vi "Smart Open.vi"(7 "Allow multiple opens?":bool=TRUE, 8 "error in (no error)":errorcluster, 10 "Channel Names":tag[](array[tag])) -> (0 "error out":errorcluster, 3 "DIO Ref Out":T1)   [LabVIEW 2021, in "DIO.lvlib"]
uses:
  <vilib>/myRIO/Instrument Drivers/Onboard IO/DIO/DIO.lvlib
  <vilib>/myRIO/Common/Instrument Driver Framework/Utilities/typedefs/Hardware Version Enum.ctl
  <vilib>/myRIO/Common/Instrument Driver Framework/Utilities/typedefs/Generic FPGA Reference.ctl
  <vilib>/myRIO/Common/Instrument Driver Framework/myRIO v1.0/DIO/typedefs/DIO Channels Enum.ctl
  <vilib>/myRIO/Common/Instrument Driver Framework/myRIO v1.0/DIO/typedefs/DIO Channels List.ctl
  <vilib>/myRIO/Instrument Drivers/Onboard IO/DIO/typedefs/DIO Reference.ctl
  <vilib>/myRIO/Common/Instrument Driver Framework/Utilities/typedefs/myRIO v1.0 Reference.ctl
  <vilib>/myRIO/Common/Instrument Driver Framework/Utilities/typedefs/myRIO Generic Hardware Reference.ctl
  <vilib>/myRIO/Instrument Drivers/Onboard IO/DIO/vis/myRIO DIO Open.xnode
  <vilib>/myRIO/Common/Instrument Driver Framework/myRIO v1.0/DIO/vis/myRIO v1.1 Open DIO.vi
  <vilib>/userdefined/High Color/nirio_resource_hc.ctl
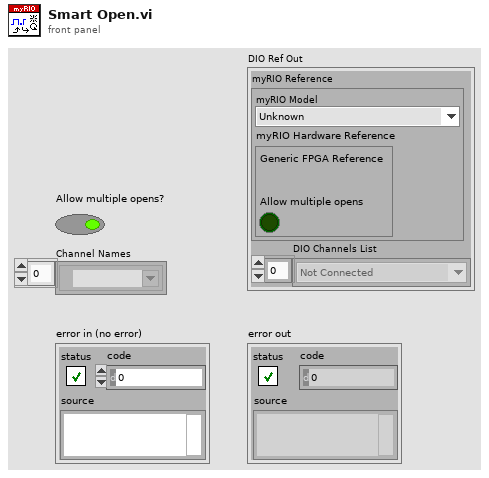
[diagram p1: front panel]
types:
  T1 = typedef "DIO.lvlib/DIO Reference.ctl" = cluster{"myRIO Reference":T2, "DIO Channels List":T6}
  T2 = typedef "myRIO Generic Hardware Reference.ctl" = cluster{"myRIO Model":T3, "myRIO Hardware Reference":T4}
  T3 = typedef "Hardware Version Enum.ctl" = enum16{"Unknown", "myRIO-1900", "myRIO-1950", "roboRIO", "NI ELVIS RIO CM", "ELVIS III"}
  T4 = typedef "myRIO v1.0 Reference.ctl" = cluster{"Generic FPGA Reference":T5, "Allow multiple opens":bool}
  T5 = typedef "Generic FPGA Reference.ctl" = refnum<k20>
  T6 = typedef "DIO Channels List.ctl" = T7[]
  T7 = typedef "DIO Channels Enum.ctl" = enum16{"Not Connected", "C/DIO0", "C/DIO1", "C/DIO2", "C/DIO3", "C/DIO4", "C/DIO5", "C/DIO6", "C/DIO7", "A/DIO0", "A/DIO1", "A/DIO2", "A/DIO3", "A/DIO4", "A/DIO5", "A/DIO6", "A/DIO7", "A/DIO8", "A/DIO9", "A/DIO10", "A/DIO11", "A/DIO12", "A/DIO13", "A/DIO14", "A/DIO15", "A/DIO16", "A/DIO17", "A/DIO18", "A/DIO19", "B/DIO0", "B/DIO1", "B/DIO2", "B/DIO3", "B/DIO4", "B/DIO5", "B/DIO6", "B/DIO7", "B/DIO8", "B/DIO9", "B/DIO10", "B/DIO11", "B/DIO12", "B/DIO13", "B/DIO14", "B/DIO15", "B/DIO16", "B/DIO17", "B/DIO18", "B/DIO19", "LED0", "LED1", "LED2", "LED3", "Button0", "DIO/DIO0", "DIO/DIO1", "DIO/DIO2", "DIO/DIO3", "DIO/DIO4", "DIO/DIO5", "DIO/DIO6", "DIO/DIO7", "DIO/DIO8", "DIO/DIO9", "SPI/CS0", "SPI/CS1", "SPI/CS2", "SPI/CS3", "LED RADIO (Green)", "LED RADIO (Red)", "LED COMM (Green)", "LED COMM (Red)", "LED MODE (Green)", "LED MODE (Red)"}
  T8 = typedef "nirio_resource_hc.ctl" = tag
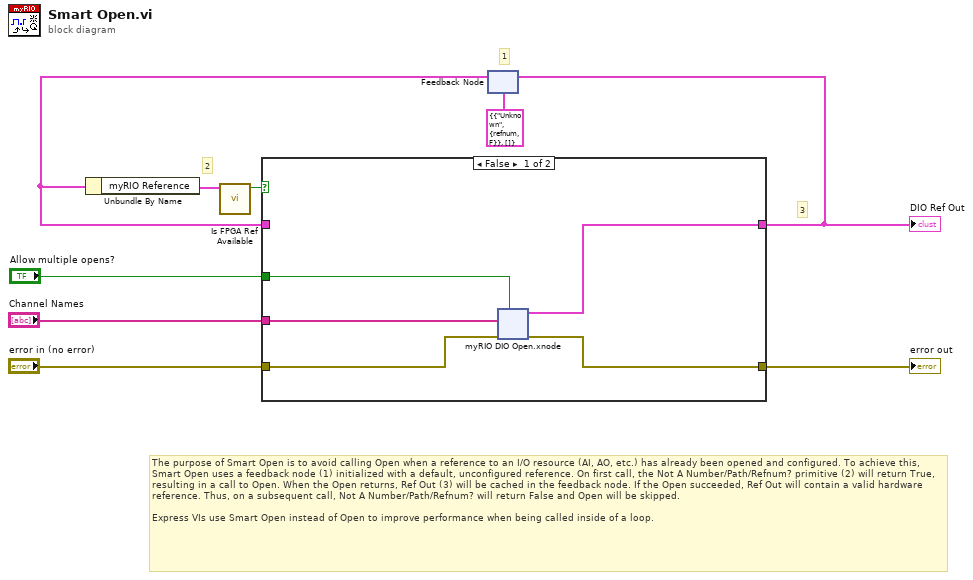
[diagram p0: block diagram]
diagram:
  # "2"
  # "1"
  # "3"
  # "The purpose of Smart Open is to avoid calling Open when a reference to an I/O resource (AI, AO, etc.) has already been opened and configured. To achieve this, Smart Open uses a feedback node (1) initialized with a default, unconfigured reference. On first call, the Not A Number/Path/Refnum? primitive (2) will return True, resulting in a call to Open. When the Open returns, Ref Out (3) will be cached in the feedback node. If the Open succeeded, Ref Out will contain a valid hardware reference. Thus, on a subsequent call, Not A Number/Path/Refnum? will return False and Open will be skipped.\n\t\nExpress VIs use Smart Open instead of Open to improve performance when being called inside of a loop."
  n1 = feedback #1(T1 {"myRIO Reference"={"myRIO Model"=enum."Unknown", "myRIO Hardware Reference"={"Generic FPGA Reference"=refnum, "Allow multiple opens"=FALSE}}, "DIO Channels List"=[]} ("AI Ref Out")) -> (w4:T1)
  n2 = Unbundle By Name(w4) -> ("myRIO Reference"=w1:T2)
  n3 = call <vilib>:"Is FPGA Ref Available.vi"("myRIO Reference"=w1) -> ("Is Available?"=w5:bool)  [unwired: 10 in]
  n4 = case shown="False" w5 {
    tunnel: "error in (no error)" -> [w14 w31]
    tunnel: [w13 w32] -> w7
    tunnel: [w12 w31] -> w8
    tunnel: w4 -> [_ w32]
    tunnel: "Allow multiple opens?" -> [w11 _]
    tunnel: "Channel Names" -> [w10 _]
    frame False {
      n5 = xnode "myRIO DIO Open.xnode"("error in (no error)"=w14, "Allow multiple opens?"=w11, "Channel Names"=w10) -> ("error out"=w12:errorcluster, "DIO Ref Out"=w13:T1)
    }
    frame True {
    }
  }
  "DIO Ref Out" <- w7
  "error out" <- w8
  n6 = feedback-in #1(w7) -> ()
